vi "Charles Rambo.vi"() -> ()   [LabVIEW 2018]
panel:
  out "Boolean":bool
  out "Gauge":dbl(knob) scale=1.0..10.0
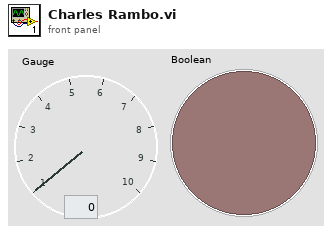
[diagram p1: front panel]
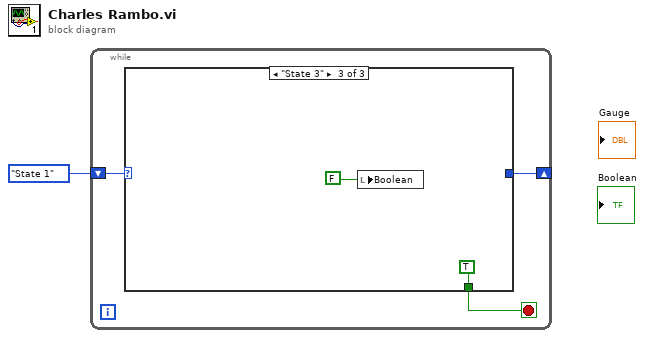
[diagram p0: block diagram]
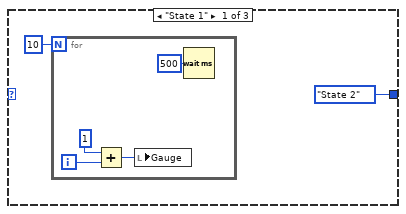
[diagram p2: hidden frame]
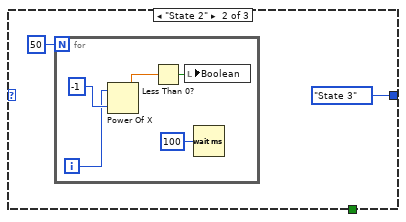
[diagram p3: hidden frame]
diagram:
  n1 = while {
    shift-right: [w3] -> _
    shift-left: enum16{"State 1", "State 2", "State 3"}."State 1" -> [w4]
    stop <- w2 stop-if-true
    n2 = case shown="\"State 3\"" w4 {
      tunnel: [enum16{"State 1", "State 2", "State 3"}."State 2" enum16{"State 1", "State 2", "State 3"}."State 3" _] -> w3
      tunnel: [_ _ TRUE] -> w2
      frame "State 1" {
        n3 = for {
          N: 10 -> [_]
          i -> [w10]
          n4 = Add(x=1, y=w10) -> (x+y=w8:i32)
          n5 = local write "Gauge"(w8) -> ()
          n6 = Wait (ms)(milliseconds to wait=500) -> ()  [unwired: 1 out]
        }
      }
      frame "State 2" {
        n7 = for {
          N: 50 -> [_]
          i -> [w13]
          n8 = Power Of X(1:-1, 2:w13) -> (0:w17:dbl)
          n9 = Less Than 0?(x=w17) -> (x < 0?=w16:bool)
          n10 = local write "Boolean"(w16) -> ()
          n11 = Wait (ms)(milliseconds to wait=u32 100) -> ()  [unwired: 1 out]
        }
      }
      frame "State 3" {
        n12 = local write "Boolean"(FALSE) -> ()
      }
    }
  }
